vi "createEventHardpointActuatorChase.vi"(8 "error in (no error)":errorcluster, 11 "UserEvents in":refnum<class "UserEvents.lvclass">) -> (0 "error out":errorcluster, 3 "UserEvents out":refnum<class "UserEvents.lvclass">)   [LabVIEW 2016, in "UserEvents.lvclass"]
uses:
  UserEvents.lvclass
  DataTypes/Topics/EventHardpointActuatorChase.ctl
  DataTypes/Topics/Parts/Timestamp.ctl
  UserEvents.lvclass/UserEvents.ctl
  DataTypes/Topics/M1M3SupportTopics.lvlib
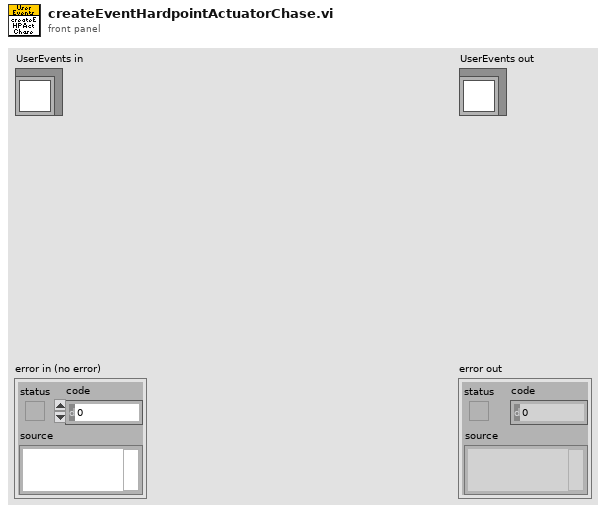
[diagram p1: front panel]
types:
  T1 = typedef "M1M3SupportTopics.lvlib/EventHardpointActuatorChase.ctl" = cluster{"Timestamp":T2, "ActuatorId":i32, "Chasing":bool}
  T2 = typedef "M1M3SupportTopics.lvlib/Timestamp.ctl" = dbl
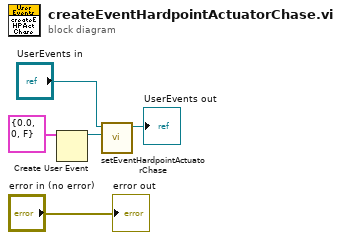
[diagram p0: block diagram]
diagram:
  n1 = Create User Event(user event datatype=T1 {"Timestamp"=0.0, "ActuatorId"=0, "Chasing"=FALSE} ("EventHardpointActuatorChase")) -> (user event=w3:refnum<user-event>)  [unwired: 1 in, 1 out]
  n2 = call "setEventHardpointActuatorChase.vi"("EventHardpointActuatorChase"=w3, "UserEvents in"="UserEvents in") -> ("UserEvents out"=→"UserEvents out":refnum<class "UserEvents.lvclass">)  [unwired: 9 in]
  "error out" <- "error in (no error)"
